vi "Project 1 LabVIEW Code.vi"() -> ()   [LabVIEW 2022 SP3]
doc: "Read one the value of one analog channel from a LINX device."
uses:
  <vilib>/MakerHub/LINX/Public/Peripherals/Analog/Analog Read 1 Chan.vi
  <vilib>/MakerHub/LINX/Public/Peripherals/Analog/Analog Read N Chans.vi
  <vilib>/MakerHub/LINX/Private/Local IO/LinxAnalogRead.vi
  <vilib>/MakerHub/LINX/Public/Utilities/Check Channel.vi
  <vilib>/MakerHub/LINX/Private/Utilties/Generate Error.vi
  <vilib>/MakerHub/LINX/LMH-LINX.lvlib
  <vilib>/ptbypt/NI_PtbyPt.lvlib
  <vilib>/Analysis/NI_AAL_SigProc.lvlib
panel:
  out "Filtered BPM":dbl[](array[numeric])
  out "BPM Range":dbl
  out "BPM Standard Deviation":dbl format="%0.2f"
  out "BPM Average":dbl format="%0.2f"
  out "Indexed Times":dbl[](array[numeric]) format="%#_6f"
  out "Amplitudes":dbl[](array[numeric])
  out "Peak-to-Peak Time (s)":dbl[](array[numeric]) caption="Peak-to-Peak Times (s)"
  out "BPM":dbl[](array[numeric])
  out "Locations":dbl[](array[numeric])
  out "# found":i32
  in  "peaks/valleys":enum32{"Peaks", "Valleys"}(ring)
  in  "threshold":dbl=3.0 format="%0.2f"
  in  "width":i32=5 min=3
  in  "Total Sample Array\ndimension size":i32=2000
  out "First Call?: T/F":bool
  out "XY Graph":cluster{dbl[], dbl[]}(graph)
  in  "PEAK DETECTION ON?":bool=TRUE
  out "Loop Time(msec)":u32
  out "mean Loop Time (msec)":dbl format="%0.2f"
  in  "AI Channel":u8
  out "Loop Rate (Hz)":dbl
  in  "Stop Button":bool
  in  "Serial Port":refnum<visa-resource-name>="COM10"
  # "Analog Read Example (Serial Interface)\n\nThis example demonstrates how to read analog input values from a LINX device connected to the host computer via Serial / USB.\n\nInstructions\n1. Select the COM Port associated with the LINX Device.\n2. Select the Analog Channel to read.\n3. Click the Run Arrow."
  # "LINX Device Settings"
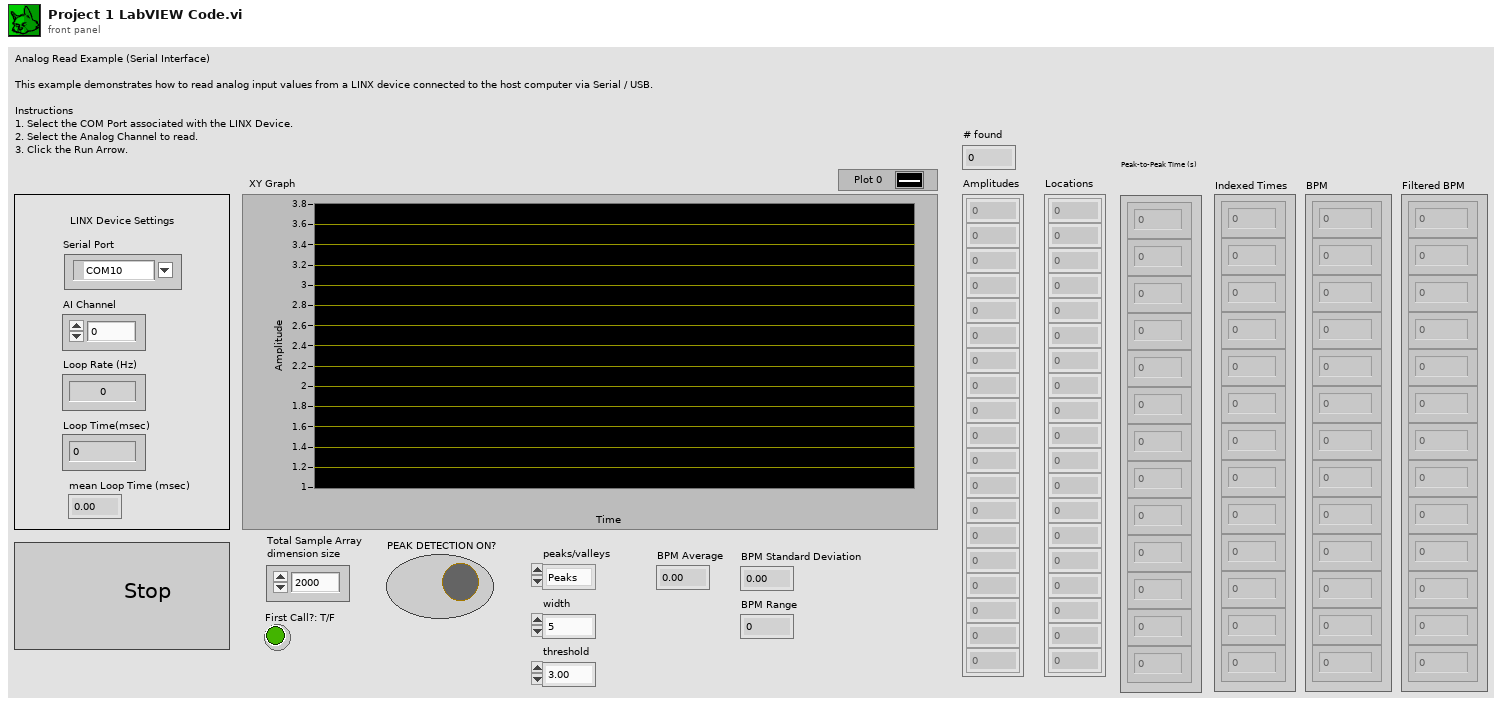
[diagram p1: front panel]
types:
  T1 = typedef "LMH-LINX.lvlib/LINX Ref.ctl" = cluster{"IO":T2, "Interface":T3, "LINX Device Config":T4}
  T2 = typedef "LMH-LINX.lvlib/Platform.ctl" = enum16{"Remote", "Local"}
  T3 = typedef "LMH-LINX.lvlib/Interface.ctl" = enum16{"Serial", "TCP"}
  T4 = typedef "LMH-LINX.lvlib/Device.lvlib/LINX Device Config.ctl" = cluster{"Interface":T3, "COM Port":refnum<visa-resource-name>, "TCP Configuration":T5, "Device Family":u8, "Device ID":u8, "Device Name":string, "TCP Ref":refnum<k5>, "Channels":T6}
  T5 = typedef "LMH-LINX.lvlib/Device.lvlib/TCP Config.ctl" = cluster{"IP Address":string, "Port":u16}
  T6 = typedef "LMH-LINX.lvlib/Channels.ctl" = cluster{"DI":u8[], "DO":u8[], "AI":u8[], "AO":u8[], "PWM":u8[], "QE":u8[], "UART":u8[], "I2C 2":u8[], "SPI":u8[], "CAN":u8[], "Servo":u8[], "AI Ref (V)":dbl, "AI Resolution (Bits)":u8, "AO Ref (V)":dbl, "AO Resolution (Bits)":u8}
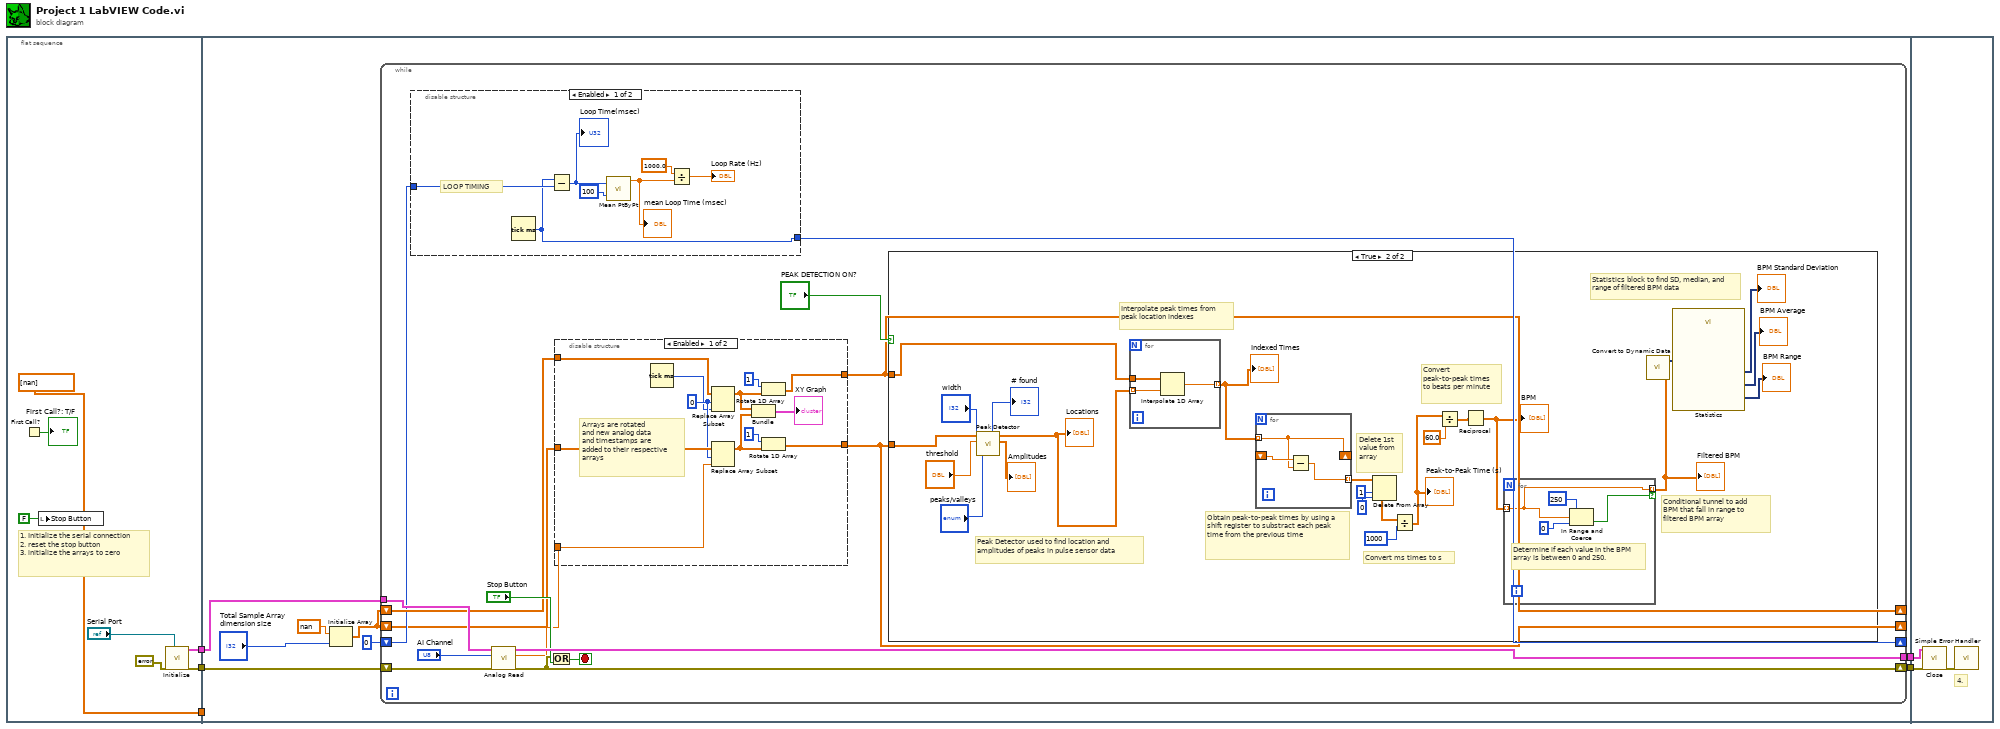
[diagram p0: block diagram]
diagram:
  n1 = flat-sequence {
    tunnel: [w9] -> w3
    tunnel: [w10] -> w2
    tunnel: [dbl[] [nan]] -> w1
    tunnel: [w18] -> w5
    tunnel: [w17] -> w4
    tunnel: w3 -> [w20]
    tunnel: w2 -> [w19]
    tunnel: w1 -> [_]
    tunnel: w5 -> [w88]
    tunnel: w4 -> [w89]
    frame #0 {
      # "1. Initialize the serial connection\n2. reset the stop button\n3. initialize the arrays to zero"
      n2 = First Call?() -> (First Call?: T/F=→"First Call?: T/F":bool)
      n3 = local write "Stop Button"(FALSE ("Stop Button")) -> ()
      n4 = call <vilib>:"Initialize.vi"("Serial Port"="Serial Port", "Error In"=errorcluster {"status"=FALSE, "code"=0, "source"=""}) -> ("Error Out"=w10:errorcluster, "LINX Resource"=w9:T1)  [unwired: 7 in, 1 out]
    }
    frame #1 {
      n5 = Initialize Array(nan ("element"), "Total Sample Array\ndimension size") -> (w15:dbl[])
      n6 = while {
        tunnel: w20 -> [w35]
        tunnel: [w33] -> w18
        shift-right: [w31] -> w17
        shift-left: w19 -> [w34]
        shift-right: [w24] -> _
        shift-left: w15 -> [w22]
        shift-right: [w26] -> _
        shift-left: u32 0 ("millisecond timer value") -> [w27]
        shift-right: [w23] -> _
        shift-left: w15 -> [w29]
        stop <- w30 stop-if-true
        n7 = disable-structure shown="Enabled" {
          disable-tunnel: w27 -> [w53 _]
          disable-tunnel: [w52 _] -> w26
          frame Enabled {
            # "LOOP TIMING"
            n8 = Tick Count (ms)() -> (millisecond timer value=w52:u32)
            n9 = Subtract(x=w52, y=w53) -> (x-y=w51:u32)
            "Loop Time(msec)" <- w51
            n10 = call <vilib>:"Mean PtByPt.vi"("x"=w51, "sample length"=100) -> ("mean"=w48:dbl)  [unwired: 2 in, 1 out]
            "mean Loop Time (msec)" <- w48
            n11 = Divide(x=1000.0, y=w48) -> (x/y=→"Loop Rate (Hz)":dbl)
          }
          frame Disabled {
          }
        }
        n12 = call-poly <vilib>:"Analog Read.vi"("Error In"=w34, "Analog Channel"="AI Channel", "LINX Resource"=w35) -> ("Error Out"=w31:errorcluster, "Voltage"=w21:dbl, "LINX Resource"=w33:T1)  [unwired: 5 in, 1 out]
        n13 = Or(x=w31, y="Stop Button") -> (x .or. y?=w30:bool)
        n14 = disable-structure shown="Enabled" {
          disable-tunnel: w29 -> [w45 _]
          disable-tunnel: w21 -> [w44 _]
          disable-tunnel: [w43 _] -> w24
          disable-tunnel: [w42 _] -> w23
          disable-tunnel: w22 -> [w38 _]
          frame Enabled {
            w37 = 0 ("index")
            # "Arrays are rotated\nand new analog data\nand timestamps are\nadded to their respective \narrays"
            n15 = Tick Count (ms)() -> (millisecond timer value=w36:u32)
            n16 = Replace Array Subset(array=w45, new element=w36, index=w37) -> (w41:dbl[])
            n17 = Replace Array Subset(array=w38, new element=w44, index=w37) -> (w40:dbl[])
            n18 = Bundle(w41, w40) -> (→"XY Graph":cluster{dbl[], dbl[]})  [unwired: 1 in]
            n19 = Rotate 1D Array(1:w41, 2:1 ("n")) -> (0:w42:dbl[])
            n20 = Rotate 1D Array(1:w40, 2:1 ("n")) -> (0:w43:dbl[])
          }
          frame Disabled {
          }
        }
        n21 = case shown="True" "PEAK DETECTION ON?" {
          tunnel: w24 -> [_ w77]
          tunnel: w23 -> [_ w70]
          frame False {
          }
          frame True {
            # "Statistics block to find SD, median, and range of filtered BPM data"
            # "Conditional tunnel to add BPM that fall in range to filtered BPM array"
            # "Convert peak-to-peak times to beats per minute"
            # "Convert ms times to s"
            # "Delete 1st value from array"
            # "Obtain peak-to-peak times by using a shift register to substract each peak time from the previous time"
            # "Interpolate peak times from peak location indexes"
            # "Peak Detector used to find location and \namplitudes of peaks in pulse sensor data"
            n22 = call <vilib>:"Peak Detector.vi"("peaks/valleys"="peaks/valleys", "width"="width", "threshold"="threshold", "X"=w77) -> ("Amplitudes"=→"Amplitudes":dbl[], "Locations"=w69:dbl[], "# found"=→"# found":i32)  [unwired: 3 in, 2 out]
            "Locations" <- w69
            n23 = for {
              tunnel: w70 -> [w87]
              tunnel: w69 -> [w86] mode=indexing
              tunnel: [w85] -> w67 mode=indexing
              n24 = Interpolate 1D Array(1:w86, 2:w87) -> (0:w85:dbl)
            }
            "Indexed Times" <- w67
            n25 = for {
              tunnel: w67 -> [w82] mode=indexing
              shift-right: [w82] -> _
              shift-left: _ -> [w83]
              tunnel: [w84] -> w64 mode=indexing
              n26 = Subtract(x=w83, y=w82) -> (x-y=w84:dbl)
            }
            n27 = Delete From Array(array=w64, length=1, index=0) -> (array with subset deleted=w61:dbl[])  [unwired: 1 out]
            n28 = Divide(x=w61, y=1000) -> (x/y=w65:dbl[])
            "Peak-to-Peak Time (s)" <- w65
            n29 = Divide(x=w65, y=60.0) -> (x/y=w71:dbl[])
            n30 = Reciprocal(x=w71) -> (1/x=w60:dbl[])
            "BPM" <- w60
            n31 = for {
              tunnel: w60 -> [w79] mode=indexing
              tunnel: [w79] -> w59 mode=indexing if=w78
              # "Determine if each value in the BPM array is between 0 and 250."
              n32 = In Range and Coerce(upper limit=250, x=w79, lower limit=0) -> (In Range?=w78:bool)  [unwired: 1 out]
            }
            "Filtered BPM" <- w59
            n33 = call "Convert to Dynamic Data"("Array"=w59) -> ("Dynamic Data Type"=w58:dynamicdata)  [unwired: 3 in]
            n34 = call "Statistics"("Signals"=w58) -> ("Median"=→"BPM Average":dynamicdata, "Standard Dev"=→"BPM Standard Deviation":dynamicdata, "Range"=→"BPM Range":dynamicdata)  [unwired: 23 in, 1 out]
          }
        }
      }
    }
    frame #2 {
      # "4."
      n35 = call <vilib>:"Close.vi"("Error In"=w89, "LINX Resource"=w88) -> ("Error Out"=w90:errorcluster)  [unwired: 9 in]
      n36 = call <vilib>:"Simple Error Handler.vi"("error in (no error)"=w90) -> ()  [unwired: 4 in, 5 out]
    }
  }
